vi "Add Row If Needed.vi"(0 "Listbox In":refnum<vi>, 1 "rings in":i32[][](array[numeric]), 2 "DefColors":u32[](array[colorbox]), 5 "Columns":T3[](array[typedef]), 7 "Default":string[](array[string]), 9 "Coords":T2, 11 "error in (no error)":errorcluster, 12 "Properties":T1) -> (3 "rings out":i32[][](array[numeric]), 4 "Listbox out":refnum<vi>, 8 "row added?":bool, 10 "Row":i32, 15 "error out":errorcluster)   [LabVIEW 2020, in "KTable.xctl"]
uses:
  KTable.xctl
  ColumnSpec.ctl
  ColumnType.ctl
  <vilib>/Utility/miscctls.llb/LVPoint32TypeDef.ctl
  Table Properties.ctl
  Array Manipulation VIs/Array-Dimensions (2D string).vi
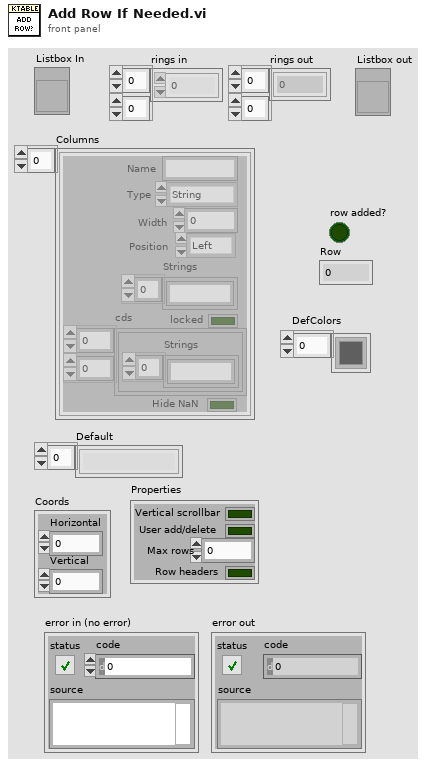
[diagram p1: front panel]
types:
  T1 = typedef "KTable.xctl/Table Properties.ctl" = cluster{"Vertical scrollbar":bool, "User add/delete":bool, "Max rows":i32, "Row headers":bool}
  T2 = typedef "LVPoint32TypeDef.ctl" = cluster{"Horizontal":i32, "Vertical":i32}
  T3 = typedef "KTable.xctl/ColumnSpec.ctl" = cluster{"Name":string, "Type":T4, "Width":i32, "Strings":string[], "Position":enum16{"Left", "Center", "Right"}, "locked":bool, "cds":cluster{"Strings":string[]}[][], "Hide NaN":bool}
  T4 = typedef "KTable.xctl/ColumnType.ctl" = enum16{"String", "Enum", "Int", "Double", "Boolean", "Ring", "Formula", "Color"}
  T5 = typedef "LVRowAndColumnTypeDef.ctl" = cluster{"Row":i32, "Column":i32}
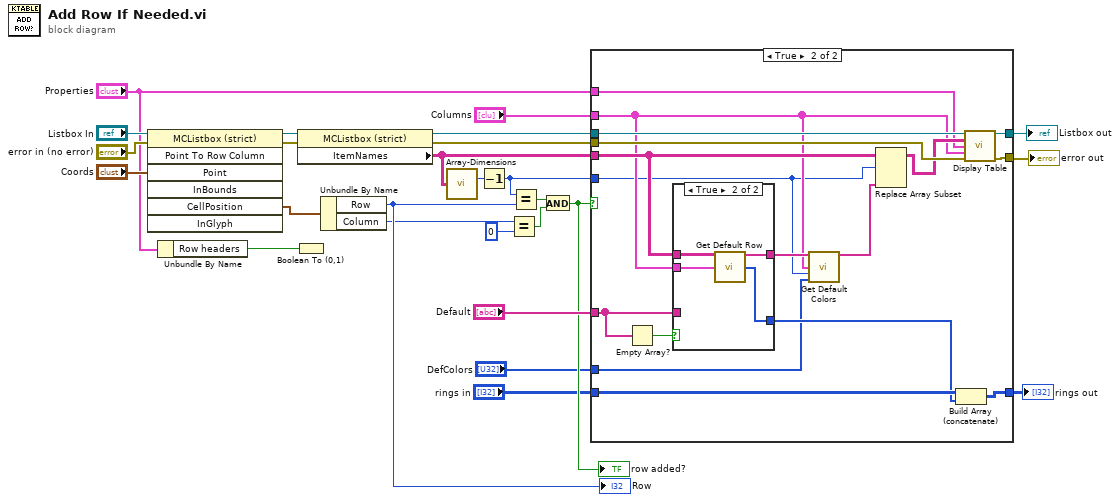
[diagram p0: block diagram]
diagram:
  n1 = invoke on="Invoke Node" class="MCListbox (strict)" method="Point To Row Column"(reference="Listbox In", error in="error in (no error)", "Point"="Coords") -> (reference out=w24:refnum<vi>, error out=w23:errorcluster, "CellPosition"=w22:T5)  [unwired: 4 in, 4 out]
  n2 = Unbundle By Name("Properties") -> ("Row headers"=w5:bool)
  n3 = Boolean To (0,1)(Boolean=w5) -> ()  [unwired: 1 out]
  n4 = property class="MCListbox (strict)"(reference=w24, error in=w23) -> (reference out=w18:refnum<vi>, error out=w17:errorcluster, "ItemNames"=w12:string[][])
  n5 = Unbundle By Name(w22) -> ("Row"=w21:i32, "Column"=w7:i32)
  "Row" <- w21
  n6 = call-poly "Array-Dimensions.vi"("2D Array"=w12) -> ("# rows"=w11:i32)  [unwired: 13 in, 1 out]
  n7 = Decrement(x=w11) -> (x-1=w10:i32)
  n8 = Equal?(x=w7, y=0) -> (x = y?=w6:bool)
  n9 = Equal?(x=w10, y=w21) -> (x = y?=w19:bool)
  n10 = And(x=w19, y=w6) -> (x .and. y?=w9:bool)
  "row added?" <- w9
  n11 = case shown="True" w9 {
    tunnel: w18 -> [w29 w44]
    tunnel: w17 -> [w28 w43]
    tunnel: [w29 w42] -> w16
    tunnel: [w28 w41] -> w15
    tunnel: "Default" -> [_ w46]
    tunnel: "Columns" -> [_ w33]
    tunnel: w12 -> [_ w40]
    tunnel: w10 -> [_ w30]
    tunnel: "Properties" -> [_ w38]
    tunnel: "rings in" -> [w27 w37]
    tunnel: [w27 w36] -> w2
    tunnel: "DefColors" -> [_ w32]
    frame False {
    }
    frame True {
      n12 = Empty Array?(array=w46) -> (empty?=w45:bool)
      n13 = case shown="True" w45 {
        tunnel: w46 -> [w47 _]
        tunnel: w40 -> [_ w51]
        tunnel: [w47 w48] -> w34
        tunnel: w33 -> [_ w49]
        tunnel: [_ w50] -> w35
        frame False {
        }
        frame True {
          n14 = call "Get Default Row.vi"("ItemNames"=w51, "Columns"=w49) -> ("Default Row"=w48:string[], "rings"=w50:i32[])  [unwired: 11 in, 1 out]
        }
      }
      n15 = call "Get Default Colors.vi"("Default Row In"=w34, "Columns"=w33, "# rows"=w30, "DefColors"=w32) -> ("Default Row Out"=w31:string[])  [unwired: 11 in]
      n16 = Replace Array Subset(array=w40, new element=w31, index (row)=w30) -> (w39:string[][])  [unwired: 1 in]
      n17 = Build Array (concatenate)(w37, w35) -> (w36:i32[][])
      n18 = call "Display Table.vi"("Listbox"=w44, "Table Items"=w39, "Properties"=w38, "Columns"=w33, "error in (no error)"=w43) -> ("reference out"=w42:refnum<vi>, "error out"=w41:errorcluster)  [unwired: 9 in]
    }
  }
  "Listbox out" <- w16
  "error out" <- w15
  "rings out" <- w2
